vi "保存配置.vi"(0 "端口号":i32=8848, 1 "等待":i32=3000, 2 "当前城市":string="荆州", 3 "手动清扫周期":dbl=2.0 min=0.1, 4 "手动清扫速度":i32=2 min=1, 5 "清扫模式选择开关":bool, 6 "晴类清扫周期":dbl=2.0 min=0.1, 7 "阴类清扫周期":dbl=2.0 min=0.1, 8 "雨类清扫周期":dbl=2.0 min=0.1, 9 "雪类清扫周期":dbl=2.0 min=0.1, 10 "沙尘类清扫周期":dbl=2.0 min=0.1, 11 "其他类清扫周期":dbl=2.0 min=0.1, 12 "晴类清扫速度":i32=1, 13 "阴类清扫速度":i32=1, 14 "雨类清扫速度":i32=1, 15 "雪类清扫速度":i32=1, 16 "沙尘类清扫速度":i32=1, 17 "其他类清扫速度":i32=1) -> ()   [LabVIEW 2016]
uses:
  <vilib>/Utility/config.llb/Write Key (I32).vi
  <vilib>/Utility/config.llb/Write Key (String).vi
  <vilib>/Utility/config.llb/Write Key (Double).vi
  <vilib>/Utility/config.llb/Write Key (Boolean).vi
  <vilib>/Utility/config.llb/NI_LVConfig.lvlib
panel:
  out "error out":errorcluster caption="错误输出"
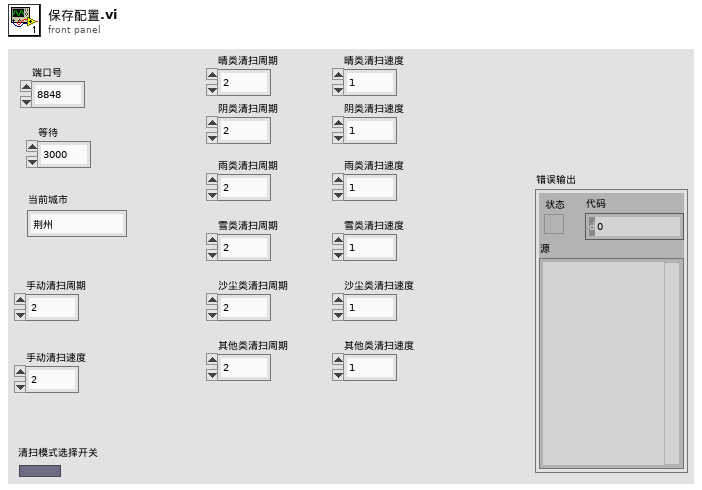
[diagram p1: front panel]
types:
  T1 = typedef "NI_LVConfig.lvlib/Config Data RefNum.ctl" = refnum<k1>
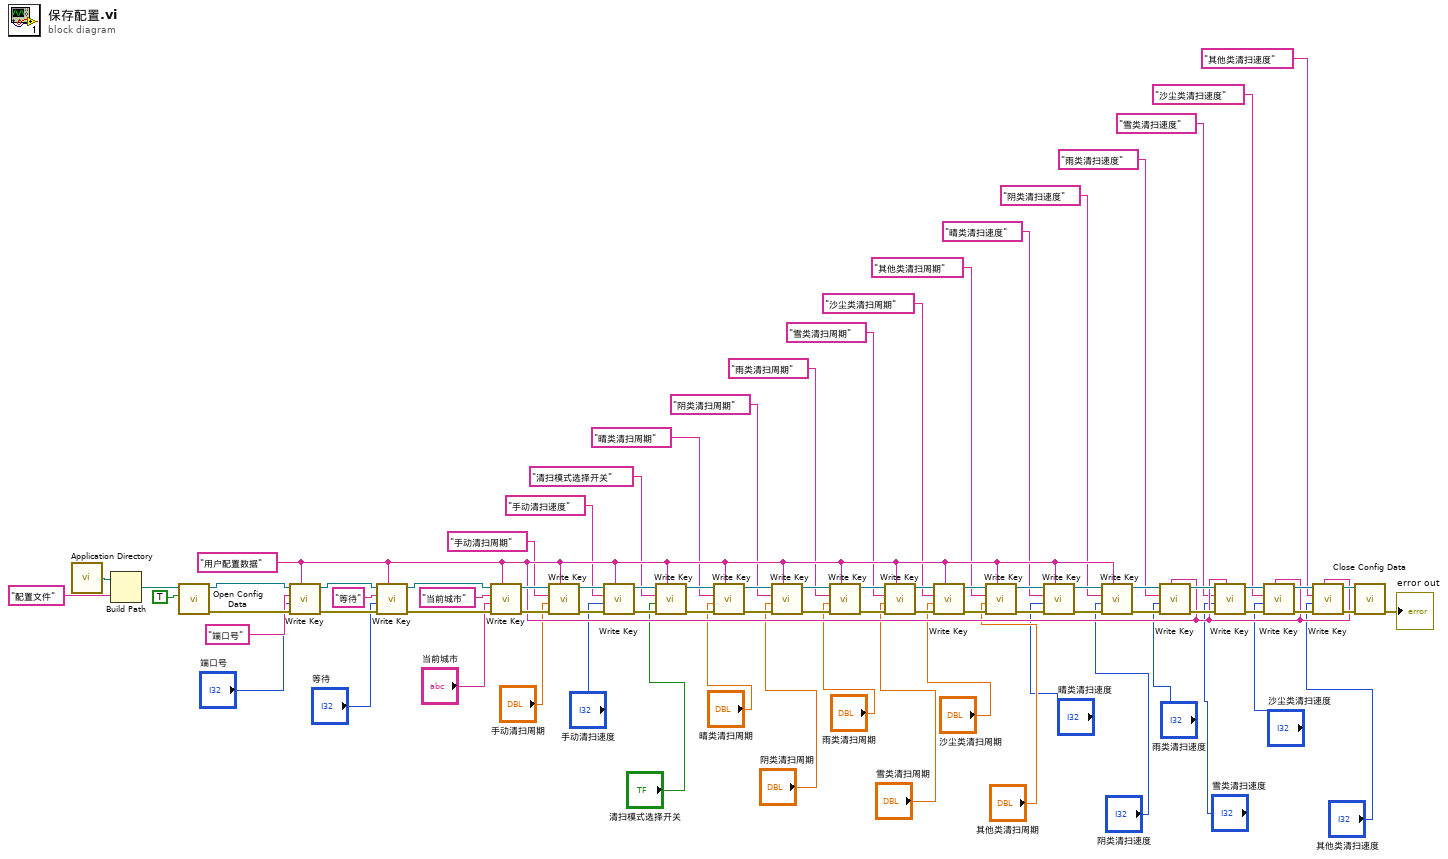
[diagram p0: block diagram]
diagram:
  w37 = "用户配置数据" ("section")
  n1 = call <vilib>:"Application Directory.vi"() -> ("Application Directory"=w79:path)
  n2 = Build Path(base path=w79, name or relative path="配置文件" ("名称或相对路径")) -> (appended path=w77:path)
  n3 = call <vilib>:"Open Config Data.vi"("create file if necessary (T)"=TRUE, "configuration file path"=w77) -> ("error out"=w75:errorcluster, "refnum"=w76:T1)  [unwired: 7 in, 1 out]
  n4 = call-poly <vilib>:"Write Key.vi"("section"=w37, "error in (no error)"=w75, "value"="端口号", "key"="端口号", "refnum"=w76) -> ("error out"=w73:errorcluster, "refnum out"=w74:T1)  [unwired: 4 in, 1 out]
  n5 = call-poly <vilib>:"Write Key.vi"("section"=w37, "error in (no error)"=w73, "value"="等待", "key"="等待", "refnum"=w74) -> ("error out"=w71:errorcluster, "refnum out"=w72:T1)  [unwired: 4 in, 1 out]
  n6 = call-poly <vilib>:"Write Key.vi"("section"=w37, "error in (no error)"=w71, "value"="当前城市", "key"="当前城市", "refnum"=w72) -> ("error out"=w69:errorcluster, "refnum out"=w70:T1)  [unwired: 4 in, 1 out]
  n7 = call-poly <vilib>:"Write Key.vi"("section"=w37, "error in (no error)"=w69, "value"="手动清扫周期", "key"="手动清扫周期", "refnum"=w70) -> ("error out"=w67:errorcluster, "refnum out"=w68:T1)  [unwired: 4 in, 1 out]
  n8 = call-poly <vilib>:"Write Key.vi"("section"=w37, "error in (no error)"=w67, "value"="手动清扫速度", "key"="手动清扫速度", "refnum"=w68) -> ("error out"=w65:errorcluster, "refnum out"=w66:T1)  [unwired: 4 in, 1 out]
  n9 = call-poly <vilib>:"Write Key.vi"("section"=w37, "error in (no error)"=w65, "value"="清扫模式选择开关", "key"="清扫模式选择开关", "refnum"=w66) -> ("error out"=w63:errorcluster, "refnum out"=w64:T1)  [unwired: 4 in, 1 out]
  n10 = call-poly <vilib>:"Write Key.vi"("section"=w37, "error in (no error)"=w63, "value"="晴类清扫周期", "key"="晴类清扫周期", "refnum"=w64) -> ("error out"=w61:errorcluster, "refnum out"=w62:T1)  [unwired: 4 in, 1 out]
  n11 = call-poly <vilib>:"Write Key.vi"("section"=w37, "error in (no error)"=w61, "value"="阴类清扫周期", "key"="阴类清扫周期", "refnum"=w62) -> ("error out"=w59:errorcluster, "refnum out"=w60:T1)  [unwired: 4 in, 1 out]
  n12 = call-poly <vilib>:"Write Key.vi"("section"=w37, "error in (no error)"=w59, "value"="雨类清扫周期", "key"="雨类清扫周期", "refnum"=w60) -> ("error out"=w51:errorcluster, "refnum out"=w58:T1)  [unwired: 4 in, 1 out]
  n13 = call-poly <vilib>:"Write Key.vi"("section"=w37, "error in (no error)"=w51, "value"="雪类清扫周期", "key"="雪类清扫周期", "refnum"=w58) -> ("error out"=w50:errorcluster, "refnum out"=w57:T1)  [unwired: 4 in, 1 out]
  n14 = call-poly <vilib>:"Write Key.vi"("section"=w37, "error in (no error)"=w50, "value"="沙尘类清扫周期", "key"="沙尘类清扫周期", "refnum"=w57) -> ("error out"=w49:errorcluster, "refnum out"=w56:T1)  [unwired: 4 in, 1 out]
  n15 = call-poly <vilib>:"Write Key.vi"("section"=w37, "error in (no error)"=w49, "value"="其他类清扫周期", "key"="其他类清扫周期", "refnum"=w56) -> ("error out"=w48:errorcluster, "refnum out"=w55:T1)  [unwired: 4 in, 1 out]
  n16 = call-poly <vilib>:"Write Key.vi"("section"=w37, "error in (no error)"=w48, "value"="晴类清扫速度", "key"="晴类清扫速度", "refnum"=w55) -> ("error out"=w47:errorcluster, "refnum out"=w54:T1)  [unwired: 4 in, 1 out]
  n17 = call-poly <vilib>:"Write Key.vi"("section"=w37, "error in (no error)"=w47, "value"="阴类清扫速度", "key"="阴类清扫速度", "refnum"=w54) -> ("error out"=w46:errorcluster, "refnum out"=w53:T1)  [unwired: 4 in, 1 out]
  n18 = call-poly <vilib>:"Write Key.vi"("section"=w37, "error in (no error)"=w46, "value"="雨类清扫速度", "key"="雨类清扫速度", "refnum"=w53) -> ("error out"=w45:errorcluster, "refnum out"=w52:T1)  [unwired: 4 in, 1 out]
  n19 = call-poly <vilib>:"Write Key.vi"("section"=w37, "error in (no error)"=w45, "value"="雪类清扫速度", "key"="雪类清扫速度", "refnum"=w52) -> ("error out"=w42:errorcluster, "refnum out"=w44:T1)  [unwired: 4 in, 1 out]
  n20 = call-poly <vilib>:"Write Key.vi"("section"=w37, "error in (no error)"=w42, "value"="沙尘类清扫速度", "key"="沙尘类清扫速度", "refnum"=w44) -> ("error out"=w41:errorcluster, "refnum out"=w43:T1)  [unwired: 4 in, 1 out]
  n21 = call-poly <vilib>:"Write Key.vi"("section"=w37, "error in (no error)"=w41, "value"="其他类清扫速度", "key"="其他类清扫速度", "refnum"=w43) -> ("error out"=w40:errorcluster, "refnum out"=w39:T1)  [unwired: 4 in, 1 out]
  n22 = call <vilib>:"Close Config Data.vi"("error in (no error)"=w40, "refnum"=w39) -> ("error out"=→"error out":errorcluster)  [unwired: 8 in, 1 out]
